vi "move_vel.vi"() -> ()   [LabVIEW 2019]
doc: "This example demonstrate how to run drive with Absolute."
uses:
  <vilib>/addons/eal4LabVIEW/ApiLib/Connection control/ealApiConnect_string.vi
  <vilib>/addons/eal4LabVIEW/eal4LabVIEW.lvlib
panel:
  in  "stop":bool
  in  "Parameters set":T1
  in  "IP address 2":string="172.17.24.131"
  # "THIAGARAJAR COLLEGE OF ENGINEERING\n      Department of Mechatronics Engineering"
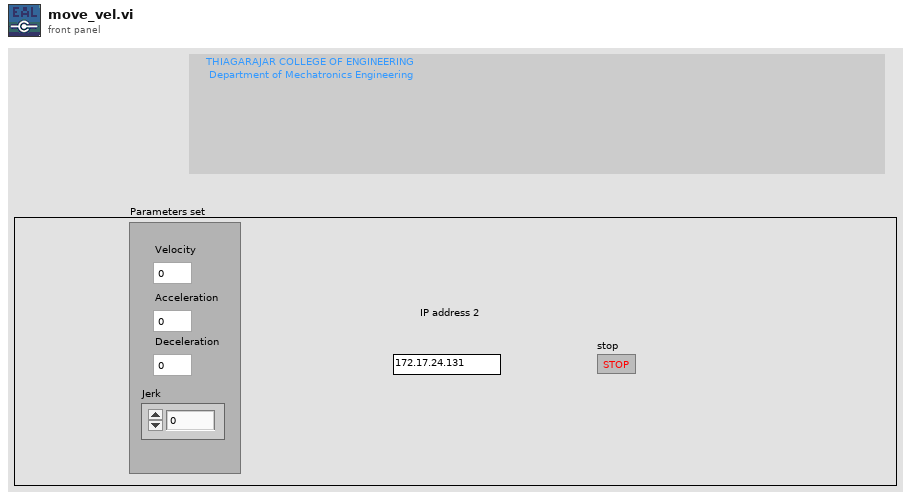
[diagram p1: front panel]
types:
  T1 = cluster{"Velocity":dbl, "Acceleration":dbl, "Deceleration":dbl, "Jerk":dbl}
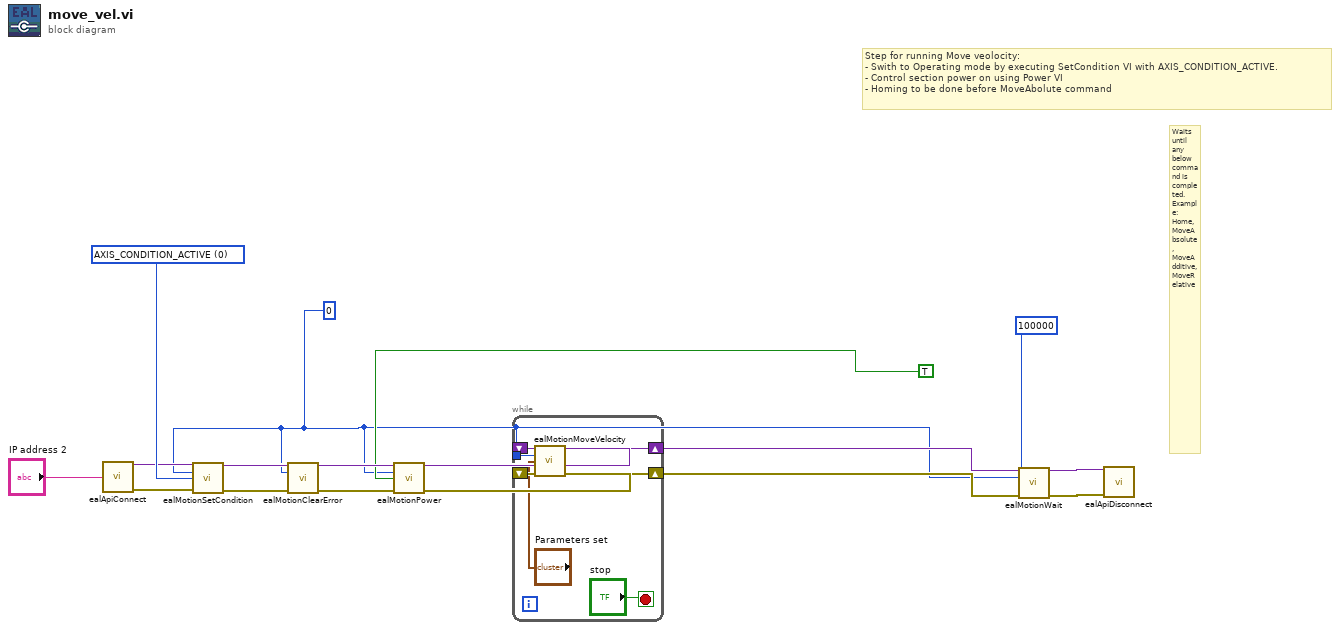
[diagram p0: block diagram]
diagram:
  w1 = 0
  w16 = 0 items=["AXIS_CONDITION_ACTIVE"=0, "AXIS_CONDITION_PARKING"=1, "AXIS_CONDITION_DEACTIVATED"=2, "AXIS_CONDITION_ACTIVE_DECOUPLED"=4, "AXIS_CONDITION_PARKING_DECOUPLED"=5, "AXIS_CONDITION_DEACTIVATED_DECOUPLED"=6, "AXIS_CONDITION_ACTIVE_PARAMETERIZATION"=8, "AXIS_CONDITION_PARKING_PARAMETERIZATION"=9, "AXIS_CONDITION_DEACTIVATED_PARAMETERIZATION"=10, "AXIS_CONDITION_ACTIVE_DECOUPLED_PARAMETERIZATION"=12, "AXIS_CONDITION_PARKING_DECOUPLED_PARAMETERIZATION"=13, "AXIS_CONDITION_DEACTIVATED_DECOUPLED_PARAMETERIZATION"=14] ("condition")
  # "Waits until any below command is completed.\nExample: Home, MoveAbsolute, MoveAdditive, MoveRelative"
  # "Step for running Move veolocity:\n- Swith to Operating mode by executing SetCondition VI with AXIS_CONDITION_ACTIVE.\n- Control section power on using Power VI\n- Homing to be done before MoveAbolute command"
  n1 = call-poly <vilib>:"ealApiConnect.vi"("ip address"="IP address 2") -> ("connection out"=w3:variant, "error out"=w2:errorcluster)  [unwired: 13 in]
  n2 = call <vilib>:"ealMotionSetCondition.vi"("connection in"=w3, "slave index"=w1, "condition"=w16, "error in (no error)"=w2) -> ("connection out"=w15:variant, "error out"=w14:errorcluster)  [unwired: 10 in]
  n3 = call <vilib>:"ealMotionClearError.vi"("connection in"=w15, "slave index"=w1, "error in (no error)"=w14) -> ("connection out"=w13:variant, "error out"=w12:errorcluster)  [unwired: 11 in]
  n4 = call <vilib>:"ealMotionPower.vi"("connection in"=w13, "slave index"=w1, "value"=TRUE, "error in (no error)"=w12) -> ("connection out"=w10:variant, "error out"=w9:errorcluster)  [unwired: 10 in]
  n5 = while {
    tunnel: w1 -> [w20]
    shift-right: [w22] -> w8
    shift-left: w10 -> [w24]
    shift-right: [w21] -> w7
    shift-left: w9 -> [w23]
    stop <- "stop" stop-if-true
    n6 = call <vilib>:"ealMotionMoveVelocity.vi"("connection in"=w24, "slave index"=w20, "parameters set"="Parameters set", "error in (no error)"=w23) -> ("connection out"=w22:variant, "error out"=w21:errorcluster)  [unwired: 10 in]
  }
  n7 = call <vilib>:"ealMotionWait.vi"("connection in"=w8, "slave index"=w1, "timeout"=100000, "error in (no error)"=w7) -> ("connection out"=w5:variant, "error out"=w4:errorcluster)  [unwired: 10 in]
  n8 = call <vilib>:"ealApiDisconnect.vi"("connection in"=w5, "error in (no error)"=w4) -> ()  [unwired: 13 in, 1 out]
